vi "LWXPS_XYZSplineVerificationResultGet.vi"(0 "XPS Reference IN":refnum<k24>, 7 "XYZ positioner Name":string, 11 "LabVIEW error IN":errorcluster) -> (2 "XPS Reference OUT":refnum<k24>, 3 "Returned error code":i32, 4 "Trajectory file name":string, 6 "Minimum position":dbl, 8 "Maximum position":dbl, 10 "Maximum velocity":dbl, 13 "LabVIEW error OUT":errorcluster, 14 "XPS Error String":string, 15 "Maximum acceleration":dbl)   [LabVIEW 2014]
uses:
  D:/XPSQ8_LabView_Library/Development/Source/Dll/Newport.XPS.CommandInterface.dll
  Dll/Newport.XPS.CommandInterface.dll
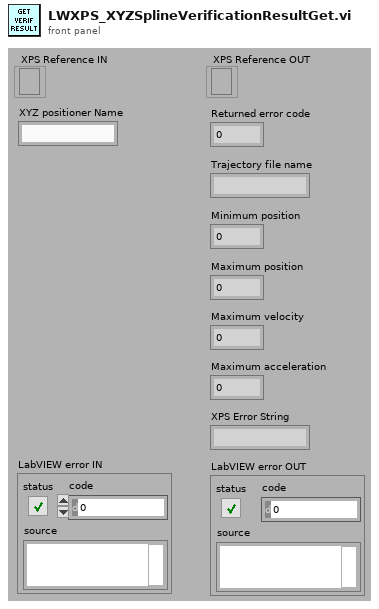
[diagram p1: front panel]
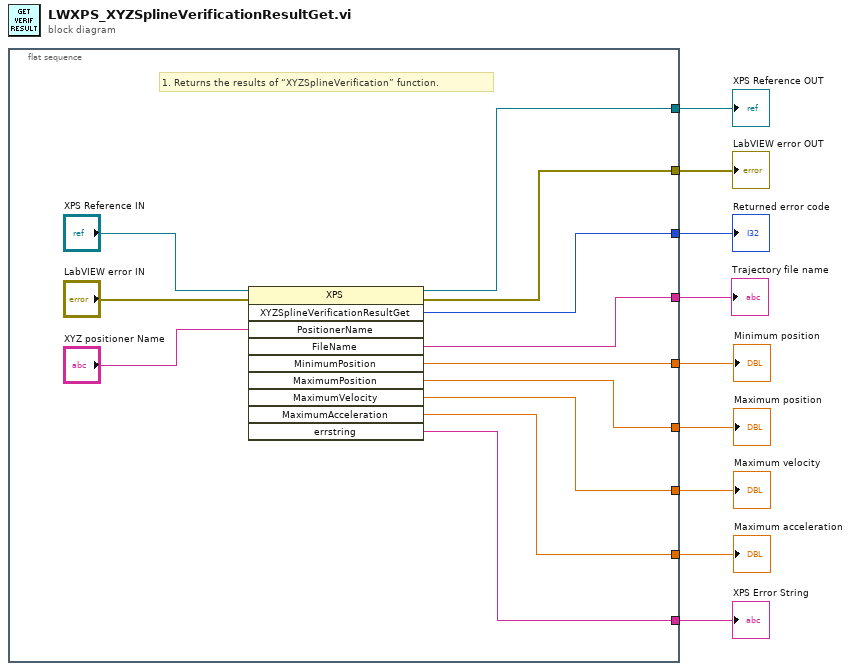
[diagram p0: block diagram]
diagram:
  n1 = flat-sequence {
    tunnel: [w15] -> w1
    tunnel: [w20] -> w9
    tunnel: [w19] -> w8
    tunnel: [w18] -> w7
    tunnel: [w14] -> w5
    tunnel: [w13] -> w4
    tunnel: [w12] -> w3
    tunnel: [w11] -> w2
    tunnel: [w10] -> w6
    frame #0 {
      # "1. Returns the results of “XYZSplineVerification” function."
      n2 = invoke class="XPS" method="XYZSplineVerificationResultGet"(reference="XPS Reference IN", error in="LabVIEW error IN", "PositionerName"="XYZ positioner Name") -> (reference out=w20:refnum<k24>, error out=w19:errorcluster, "XYZSplineVerificationResultGet"=w18:i32, "FileName"=w15:string, "MinimumPosition"=w14:dbl, "MaximumPosition"=w13:dbl, "MaximumVelocity"=w12:dbl, "MaximumAcceleration"=w11:dbl, "errstring"=w10:string)  [unwired: 7 in, 1 out]
    }
  }
  "XPS Error String" <- w6
  "XPS Reference OUT" <- w9
  "LabVIEW error OUT" <- w8
  "Returned error code" <- w7
  "Minimum position" <- w5
  "Maximum position" <- w4
  "Maximum velocity" <- w3
  "Maximum acceleration" <- w2
  "Trajectory file name" <- w1
